vi "Write AO.vi"(8 "error in (no error)":errorcluster, 10 "AO []":waveform(dbl)[](array[waveform]), 11 "DAQmx in":refnum<class "DAQmx.lvclass">) -> (0 "error out":errorcluster, 2 "AO out []":waveform(dbl)[](array[waveform]), 3 "DAQmx out":refnum<class "DAQmx.lvclass">, 4 "AO time (ms)":u32=53)   [LabVIEW 2019, in "DAQmx.lvclass"]
uses:
  DAQmx.lvclass
  DAQmx.lvclass/DAQmx.ctl
  <vilib>/DAQmx/write.llb/DAQmx Write (Analog 1D Wfm NChan NSamp).vi
  <vilib>/Waveform/WDTOps.llb/WDT Append Waveforms DBL.vi
  <vilib>/DAQmx/miscellaneous.llb/DAQmx Fill In Error Info.vi
  Instrument.DAQ/Instrument.DAQ.lvclass
panel:
  in  "show graph":bool
  out "AO (previous)":waveform(dbl)[](array[waveform])
  out "Waveform Graph":waveform(dbl)[](graph)
  out "P Check":bool[](array[boolean])
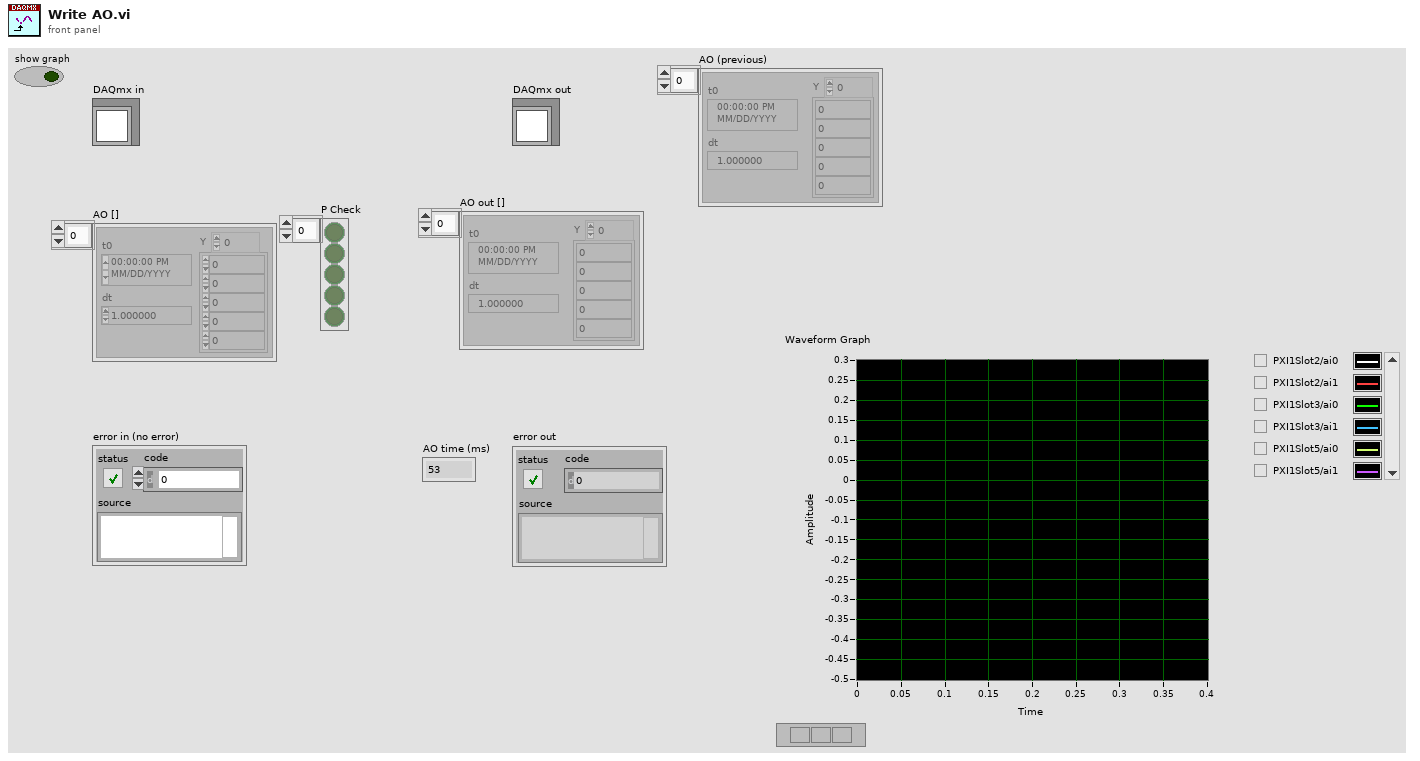
[diagram p1: front panel]
types:
  T1 = typedef "DAQmx.lvclass/DAQ.Config.Device Type--enum.ctl" = enum16{"None", "USB-4431", "PXI-446x"}
  T2 = typedef "DAQmx.lvclass/DAQ.Config.AO--Cluster--Array.ctl" = T3[]
  T3 = typedef "DAQmx.lvclass/DAQ.Config.AO--Cluster.ctl" = cluster{"Channels":tag, "Range":T4, "output terminal configuration":i32, "Type":T1}
  T4 = typedef "DAQmx.lvclass/DAQ.Config.AO.Range--enum.ctl" = enum16{"±0.1", "±1.0", "±10.0", ""}
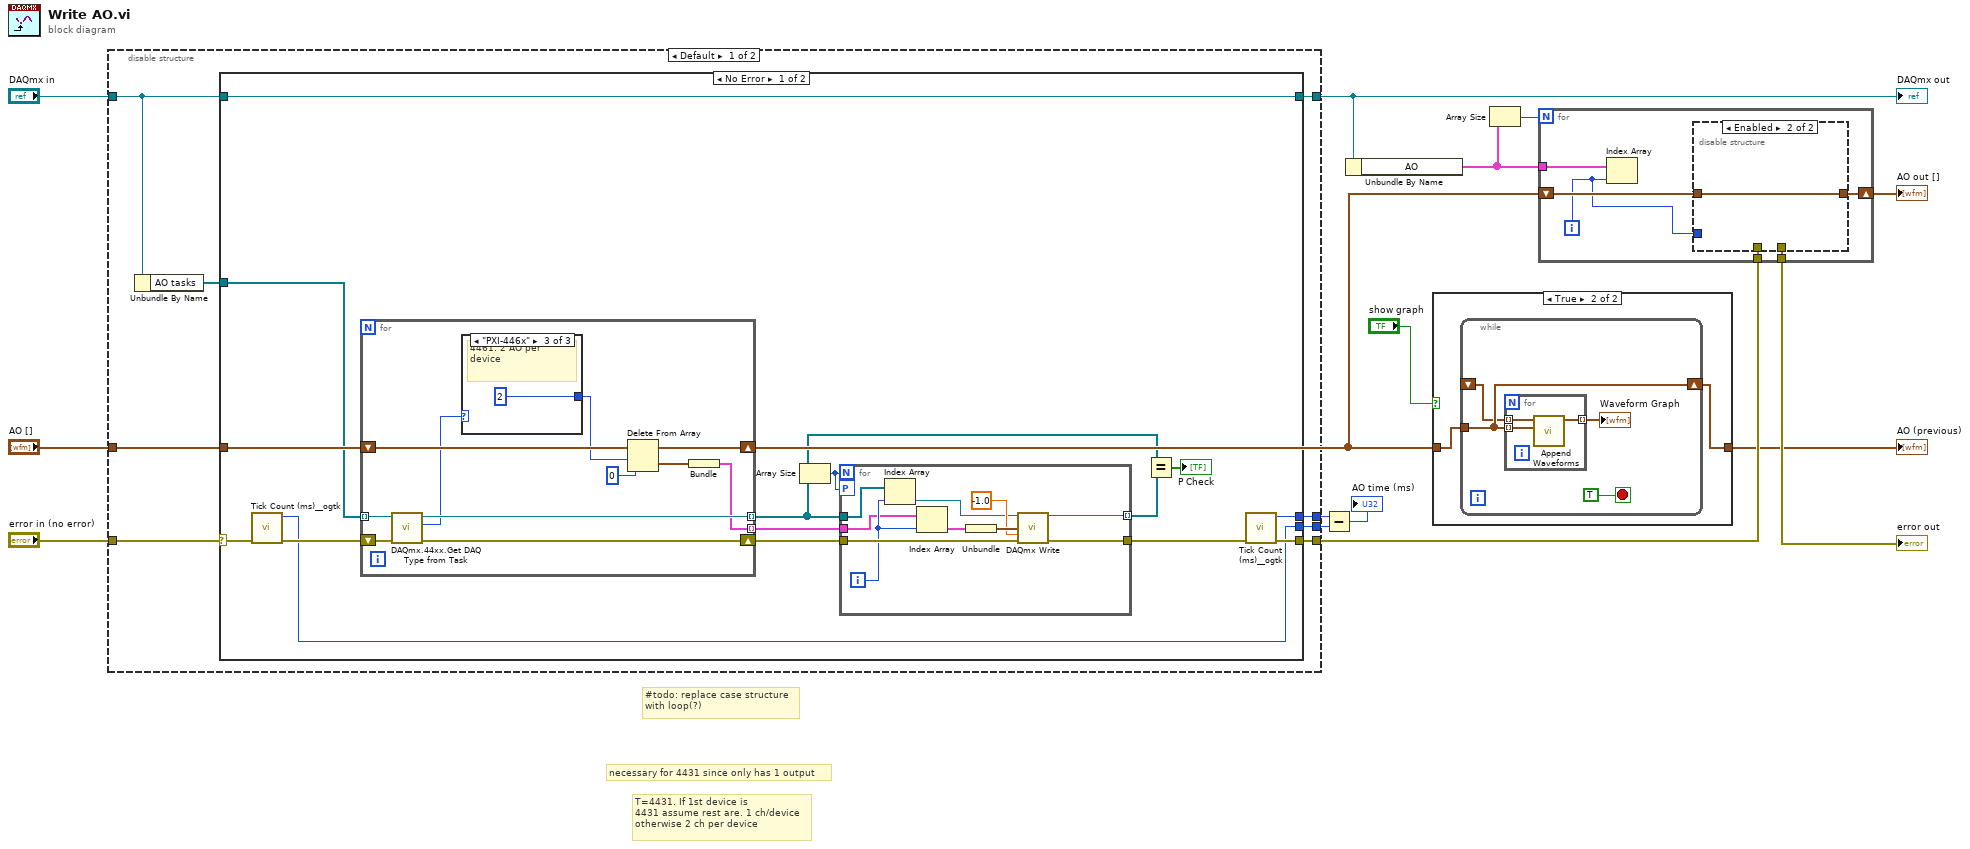
[diagram p0: block diagram]
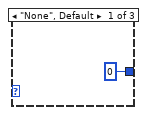
[diagram p2: hidden frame]
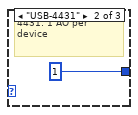
[diagram p3: hidden frame]
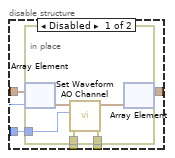
[diagram p7: hidden frame]
diagram:
  # "#todo: replace case structure\nwith loop(?)"
  # "T=4431. If 1st device is \n4431 assume rest are. 1 ch/device\notherwise 2 ch per device"
  # "necessary for 4431 since only has 1 output"
  n1 = disable-structure shown="Default" {
    disable-tunnel: [w22 w65] -> w8
    disable-tunnel: "DAQmx in" -> [w20 w64]
    disable-tunnel: "AO []" -> [w21 _]
    disable-tunnel: "error in (no error)" -> [w15 w65]
    disable-tunnel: [w19 w64] -> w1
    disable-tunnel: [w18 _] -> w14
    disable-tunnel: [w17 _] -> w11
    frame condition #0 (active) {
      n2 = Unbundle By Name(w20) -> ("AO tasks"=w16:refnum<k21>[])
      n3 = case shown="No Error" w15 {
        selector: w15 -> [w31 w62]
        tunnel: [w34 w62] -> w22
        tunnel: w21 -> [w36 _]
        tunnel: w16 -> [w37 _]
        tunnel: w20 -> [w32 w63]
        tunnel: [w32 w63] -> w19
        tunnel: [w33 _] -> w18
        tunnel: [w29 _] -> w17
        frame No Error {
          n4 = call <userlib>:"Tick Count (ms)__ogtk.vi"("error in (no error)"=w31) -> ("error out"=w30:errorcluster, "millisecond timer value"=w29:u32)  [unwired: 9 in]
          n5 = for {
            tunnel: [w38] -> w27 mode=indexing
            shift-right: [w47] -> w28
            shift-left: w30 -> [w48]
            tunnel: w37 -> [w46] mode=indexing
            shift-right: [w45] -> _
            shift-left: w36 -> [w43]
            tunnel: [w44] -> w26 mode=indexing
            n6 = call "DAQmx.44xx.Get DAQ Type from Task.vi"("error in (no error)"=w48, "Task in"=w46) -> ("error out"=w47:errorcluster, "DAQ Type"=w42:T1, "Task out"=w44:refnum<k21>)  [unwired: 6 in, 1 out]
            n7 = case shown="\"PXI-446x\"" w42 {
              tunnel: [0 ("length") 1 ("length") 2 ("length")] -> w39
              frame "None", Default {
              }
              frame "USB-4431" {
                # "4431: 1 AO per device"
              }
              frame "PXI-446x" {
                # "4461: 2 AO per device"
              }
            }
            n8 = Delete From Array(array=w43, length=w39, index=0) -> (deleted portion=w41:waveform(dbl)[], array with subset deleted=w45:waveform(dbl)[])
            n9 = Bundle("AO []"=w41) -> (w38:cluster{"AO []":waveform(dbl)[]})  [unwired: 1 in]
          }
          n10 = Array Size(array=w26) -> (size(s)=w24:i32)
          n11 = for {
            N: w24 -> [_]
            tunnel: w26 -> [w54]
            tunnel: w27 -> [w55]
            tunnel: w28 -> [w61]
            tunnel: [w52] -> w35
            workers-P: w24 -> [_]
            tunnel: [w53] -> w23 mode=indexing
            i -> [w56]
            n12 = Index Array(array=w54, index=w56) -> (element=w57:refnum<k21>)
            n13 = Index Array(array=w55, index=w56) -> (element=w58:cluster{"AO []":waveform(dbl)[]})
            n14 = Unbundle(w58) -> ("AO []"=w60:waveform(dbl)[])
            n15 = call-poly <vilib>:"DAQmx Write.vi"("task/channels in"=w57, "data"=w60, "timeout"=-1.0, "error in"=w61) -> ("task out"=w53:refnum<k21>, "error out"=w52:errorcluster)  [unwired: 9 in, 1 out]
          }
          n16 = Equal?(x=w26, y=w23) -> (x = y?=→"P Check":bool[])
          n17 = call <userlib>:"Tick Count (ms)__ogtk.vi"("error in (no error)"=w35) -> ("error out"=w34:errorcluster, "millisecond timer value"=w33:u32)  [unwired: 9 in]
        }
        frame Error {
        }
      }
    }
    frame condition #1 {
    }
  }
  "DAQmx out" <- w1
  n18 = Subtract(x=w14, y=w11) -> (x-y=→"AO time (ms)":u32)
  n19 = Unbundle By Name(w1) -> ("AO"=w4:T2)
  n20 = case shown="True" "show graph" {
    tunnel: "AO []" -> [w66 w67]
    tunnel: [w66 w68] -> w2
    frame False {
    }
    frame True {
      n21 = while {
        shift-right: [w70] -> w68
        shift-left: _ -> [w69]
        tunnel: w67 -> [w70]
        stop <- TRUE stop-if-true
        n22 = for {
          tunnel: [w75] -> w71 mode=indexing
          tunnel: w69 -> [w74] mode=indexing
          tunnel: w70 -> [w73] mode=indexing
          n23 = call-poly <vilib>:"Append Waveforms.vi"("waveform B"=w73, "waveform A"=w74) -> ("waveform out"=w75:waveform(dbl))  [unwired: 8 in, 1 out]
        }
        "Waveform Graph" <- w71
      }
    }
  }
  "AO (previous)" <- w2
  n24 = Array Size(array=w4) -> (size(s)=w5:i32)
  n25 = for {
    N: w5 -> [_]
    tunnel: w8 -> [w80]
    tunnel: [w79] -> w7
    shift-right: [w78] -> w9
    shift-left: "AO []" -> [w81]
    tunnel: w4 -> [w77]
    i -> [w76]
    n26 = Index Array(array=w77, index=w76) -> ()  [unwired: 1 out]
    n27 = disable-structure shown="Enabled" {
      disable-tunnel: w81 -> [w86 w92]
      disable-tunnel: w80 -> [w85 _]
      disable-tunnel: [w84 _] -> w79
      disable-tunnel: [w83 w92] -> w78
      disable-tunnel: w76 -> [w82 _]
      frame Disabled {
        n28 = in-place {
          in-place-border: w85 -> [w89]
          in-place-border: [w88] -> w84
          in-place-border: w82 -> [w87]
          n29 = in-place-array #1(w86, w82) -> (w91:waveform(dbl))
          n30 = call "Set Waveform AO Channel.vi"("error in (no error)"=w89, "AO Channel"=w87, "Waveform in"=w91) -> ("error out"=w88:errorcluster, "Waveform out"=w90:waveform(dbl))  [unwired: 7 in]
          n31 = in-place-array #1(w90) -> (w83:waveform(dbl)[])  [unwired: 1 out]
        }
      }
      frame Enabled {
      }
    }
  }
  "error out" <- w7
  "AO out []" <- w9
